vi "test_LogFile Exists on RT cRIO.vi"(8 "error in (no error)":errorcluster, 11 "TestCase in":refnum<class "TLCD System Tests.lvclass">) -> (0 "error out":errorcluster, 3 "TestCase out":refnum<class "TLCD System Tests.lvclass">)   [LabVIEW 2019, in "TLCD System Tests.lvclass"]
uses:
  TLCD System Tests.lvclass
  <vilib>/addons/_JKI Toolkits/VI Tester/TestCase.llb/TestCase.lvclass
  TLCD Test Class/TLCD Test Class.lvclass
  4c642fb7-04a0-4729-a002-4e235dd1b0d8.vi
  C:/Program Files (x86)/National Instruments/LabVIEW 2019/vi.lib/addons/_JKI Toolkits/VI Tester/TestCase.llb/TestCase.lvclass
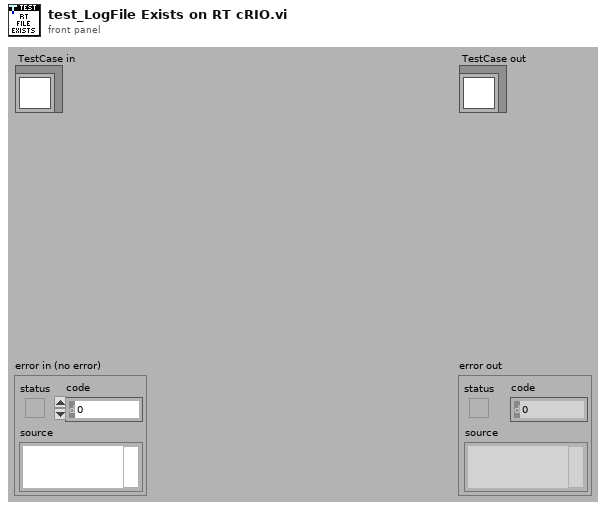
[diagram p1: front panel]
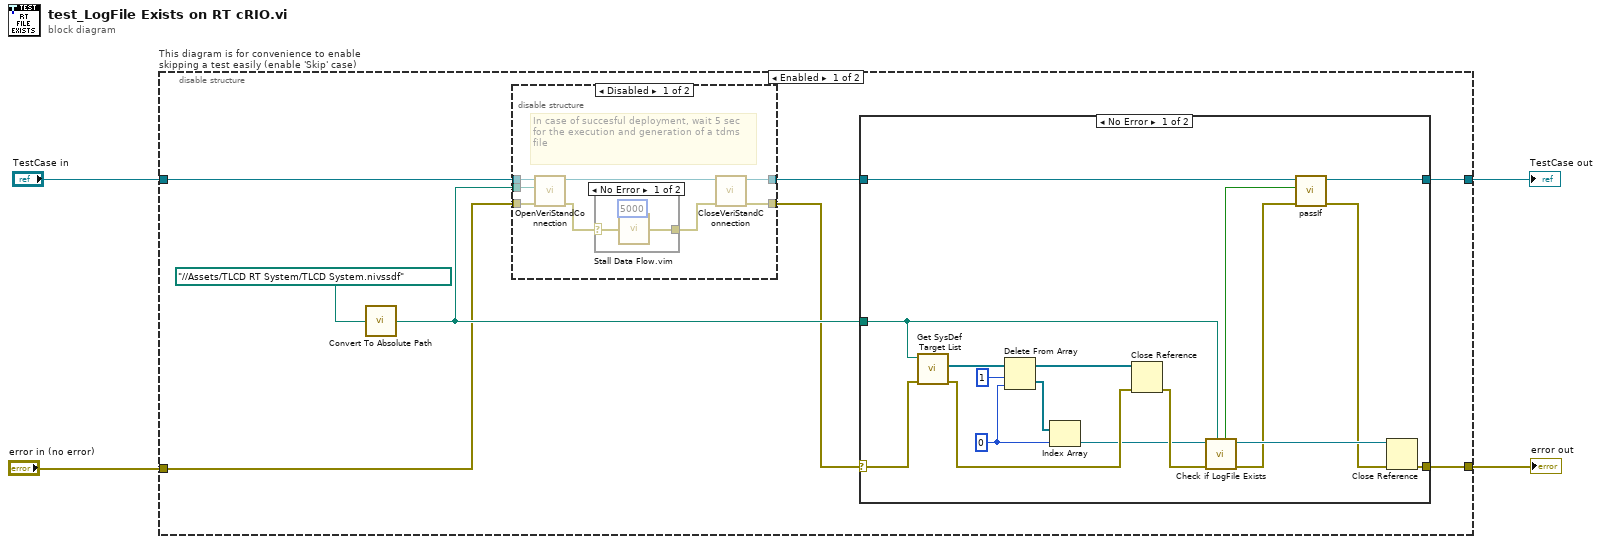
[diagram p0: block diagram]
diagram:
  n1 = disable-structure "This diagram is for convenience to enable skipping a test easily (enable 'Skip' case)" shown="Enabled" {
    disable-tunnel: "TestCase in" -> [w9 w49]
    disable-tunnel: [w10 w47] -> w1
    disable-tunnel: [w11 w48] -> w3
    disable-tunnel: "error in (no error)" -> [w6 w46]
    frame Enabled {
      n2 = call "Convert To Absolute Path.vi"("System Definition File Path"=path "../../Assets/TLCD RT System/TLCD System.nivssdf" ("relative base path")) -> ("Absolute path"=w7:path)
      n3 = disable-structure shown="Disabled" {
        disable-tunnel: w9 -> [w17 w26]
        disable-tunnel: [w16 w26] -> w8
        disable-tunnel: w7 -> [w15 _]
        disable-tunnel: w6 -> [w14 w25]
        disable-tunnel: [w13 w25] -> w5
        frame Disabled {
          # "In case of succesful deployment, wait 5 sec for the execution and generation of a tdms file"
          n4 = call-dynamic "OpenVeriStandConnection.vi"("error in (no error)"=w14, "System Definition File"=w15, "VeriStand Test Case in"=w17) -> ("error out"=w19:errorcluster, "VeriStand Test Case out"=w20:refnum<class "TLCD System Tests.lvclass">)  [unwired: 6 in, 1 out]
          n5 = case shown="No Error" w19 {
            selector: w19 -> [w23 w24]
            tunnel: [w21 w24] -> w18
            frame No Error {
              n6 = call "Stall Data Flow.vim"("value in"=w23, "milliseconds to wait"=u32 5000) -> ("value out"=w21:errorcluster)  [unwired: 1 out]
            }
            frame Error {
            }
          }
          n7 = call-dynamic "CloseVeriStandConnection.vi"("error in (no error)"=w18, "VeriStand Test Case in"=w20) -> ("error out"=w13:errorcluster, "VeriStand Test Case out"=w16:refnum<class "TLCD System Tests.lvclass">)  [unwired: 8 in]
        }
        frame Enabled {
          # "Deployment currenctly does\nnot work for Linux_x64 targets, however there is an already pregenerated file available on RT"
        }
      }
      n8 = case shown="No Error" w5 {
        selector: w5 -> [w27 w45]
        tunnel: [w43 w45] -> w11
        tunnel: [w33 w44] -> w10
        tunnel: w8 -> [w29 w44]
        tunnel: w7 -> [w28 _]
        frame No Error {
          w39 = 0 ("index")
          n9 = call "Get SysDef Target List.vi"("error in (no error)"=w27, "System Definition Path"=w28) -> ("error out"=w37:errorcluster, "Target List"=w42:refnum<k24>[])  [unwired: 8 in]
          n10 = Delete From Array(array=w42, length=1, index=w39) -> (deleted portion=w40:refnum<k24>[], array with subset deleted=w38:refnum<k24>[])
          n11 = Index Array(array=w40, index=w39) -> (element=w34:refnum<k24>)
          n12 = Close Reference(reference=w38, error in (no error)=w37) -> (error out=w35:errorcluster)
          n13 = call "Check if LogFile Exists.vi"("System Definition Path"=w28, "error in (no error)"=w35, "Target Refnum in"=w34) -> ("error out"=w32:errorcluster, "Target Refnum out"=w36:refnum<k24>, "LogFile Exists?"=w30:bool)  [unwired: 6 in]
          n14 = call-dynamic "passIf.vi"("error in (no error)"=w32, "pass"=w30, "TestCase in"=w29) -> ("error out"=w31:errorcluster, "TestCase out"=w33:refnum<class "TLCD System Tests.lvclass">)  [unwired: 7 in]
          n15 = Close Reference(reference=w36, error in (no error)=w31) -> (error out=w43:errorcluster)
        }
        frame Error {
        }
      }
    }
    frame Disabled {
      # "skip test result while test is under development"
      n16 = call <vilib>:"skip.vi"("error in (no error)"=w46, "TestCase in"=w49) -> ("error out"=w48:errorcluster, "TestCase out"=w47:refnum<class "TLCD System Tests.lvclass">)  [unwired: 8 in]
    }
  }
  "error out" <- w3
  "TestCase out" <- w1
